vi "DLTS - timing calculation (time window) (SubVI).vi"(0 "Time window":dbl[unit]=100.0 format="%#.1p", 1 "Sampling rate":dbl(ring)=107142.859375 items=["13 kSa"=13392.857422, "27 kSa"=26785.714844, "54 kSa"=53571.429687, "107 kSa"=107142.859375], 2 "Averaging":i32=1, 3 "1st pulse duration":dbl[unit]=100.0 format="%#.1p", 4 "2nd pulse duration":dbl[unit]=100.0 format="%#.1p", 5 "Acquisition delay":dbl[unit]=1.0 min=0.0 max=1.0 step=1e-06 format="%#_6p", 6 "2 pulse mode":bool) -> (14 "Number of samples":i32, 15 "Acquisition duration":dbl[unit], 16 "Pulse off time":dbl[unit])   [LabVIEW 2019]
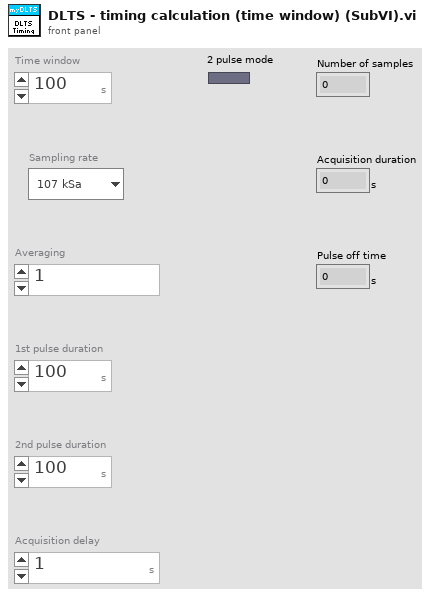
[diagram p1: front panel]
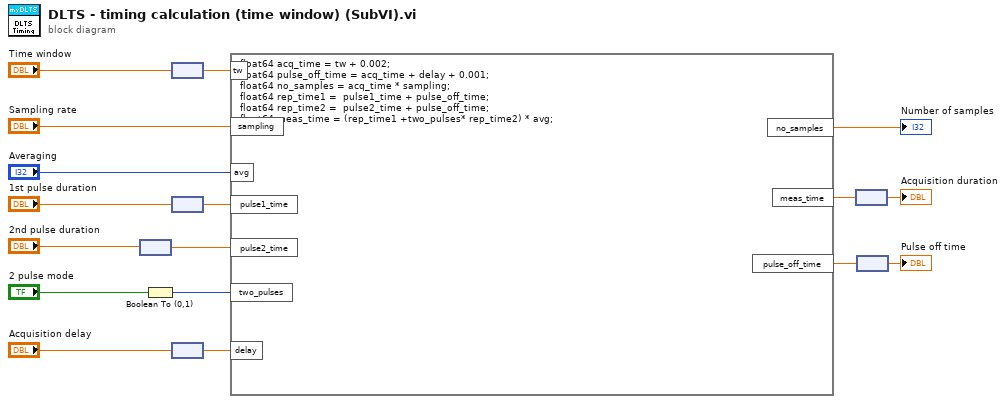
[diagram p0: block diagram]
diagram:
  n1 = node("2nd pulse duration") -> (w3:dbl)
  n2 = Boolean To (0,1)(Boolean="2 pulse mode") -> (0, 1=w1:i16)
  n3 = node("Time window") -> (w16:dbl)
  n4 = node("1st pulse duration") -> (w17:dbl)
  n5 = node("Acquisition delay") -> (w15:dbl)
  n6 = formula code="float64 acq_time = tw + 0.002;\nfloat64 pulse_off_time = acq_time + delay + 0.001;\nfloat64 no_samples = acq_time * sampling;\nfloat64 rep_time1 =  pulse1_time + pulse_off_time;\nfloat64 rep_time2 =  pulse2_time + pulse_off_time;\nfloat64 meas_time = (rep_time1 +two_pulses* rep_time2) * avg;"("tw"=w16, "sampling"="Sampling rate", "pulse1_time"=w17, "avg"="Averaging", "delay"=w15, "pulse2_time"=w3, "two_pulses"=w1) -> ("no_samples"=→"Number of samples":dbl, "meas_time"=w10:dbl, "pulse_off_time"=w8:dbl)
  n7 = node(w10) -> (→"Acquisition duration":dbl[unit])
  n8 = node(w8) -> (→"Pulse off time":dbl[unit])
